vi "Dead Reckoning.vi"(8 "Path":dbl[](array[numeric]), 9 "Yaw angle":dbl, 10 "Channel 6 position":u8, 11 "Velocity":dbl) -> (0 "Yaw with offset":dbl, 1 "Reference yaw":dbl, 2 "Run dead reckoning?":bool, 3 "Reference lean":dbl, 4 "case":dbl)   [LabVIEW 2016]
uses:
  <vilib>/Simulation/Shared/_Datatypes/SIM SISO Transfer Function.ctl
  <vilib>/Simulation/DiscreteLinear/Implementation/NILVSim Discrete Transfer Function Direct.llb/SIM Discrete Transfer Function Diagram (SISO).vi
  <vilib>/Simulation/ContinuousLinear/Implementation/Shared/SIM Transfer Function Support.llb/SIM TransferFunction Normalize to Buffer.vi
  <vilib>/Simulation/DiscreteLinear/Implementation/Shared/SIM Init Discrete States.vi
  <vilib>/Simulation/DiscreteLinear/Implementation/NILVSim Discrete Transfer Function Direct.llb/SIM Transfer Function Direct core (SISO).vi
  <vilib>/Simulation/ContinuousLinear/Implementation/Shared/SIM Transfer Function Support.llb/SIM TransferFunction Normalize.vi
  <vilib>/Simulation/Implementation/Shared/SIM Polynomials.llb/SIM Remove Zero Coefficients (DBL).vi
  <vilib>/Simulation/Implementation/Shared/SIM Polynomials.llb/SIM Divide Polynomials (DBL).vi
  <vilib>/Simulation/Implementation/Shared/SIM BuildSimErr.vi
  <vilib>/Simulation/Implementation/XNodeFramework/SimXNode/SimX.xnode
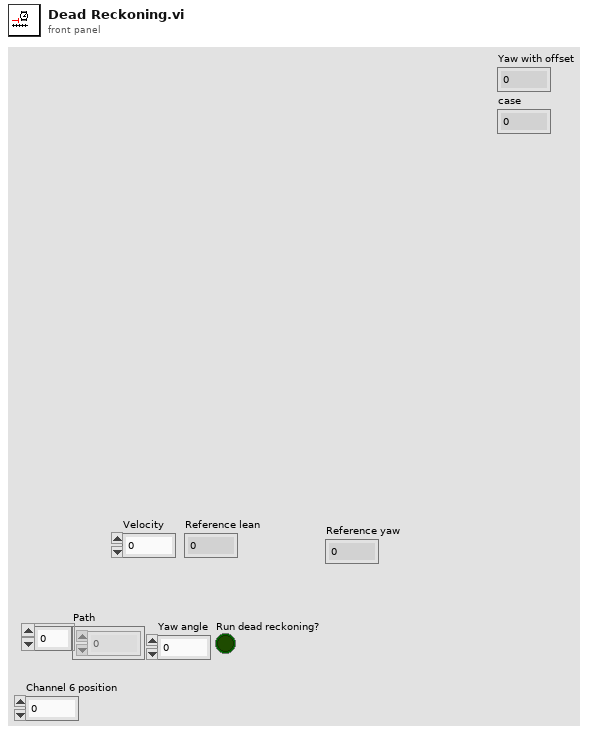
[diagram p1: front panel]
types:
  T1 = cluster{"proportional gain (Kc)":dbl, "integral time (Ti, min)":dbl, "derivative time (Td, min)":dbl}
  T2 = typedef "SIM SISO Transfer Function.ctl" = cluster{"Numerator":dbl[], "Denominator":dbl[]}
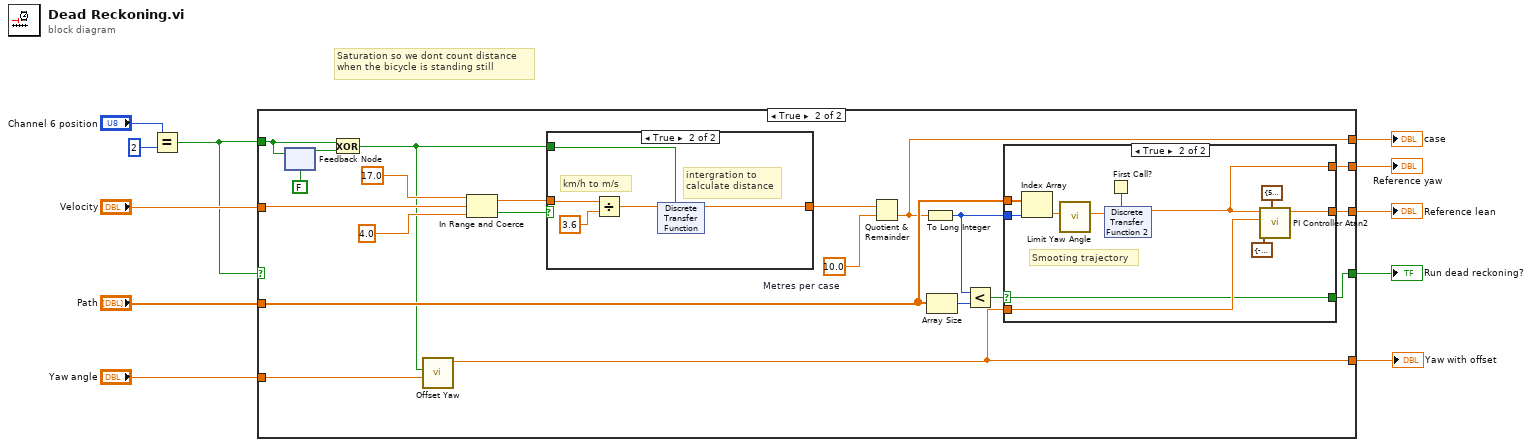
[diagram p0: block diagram]
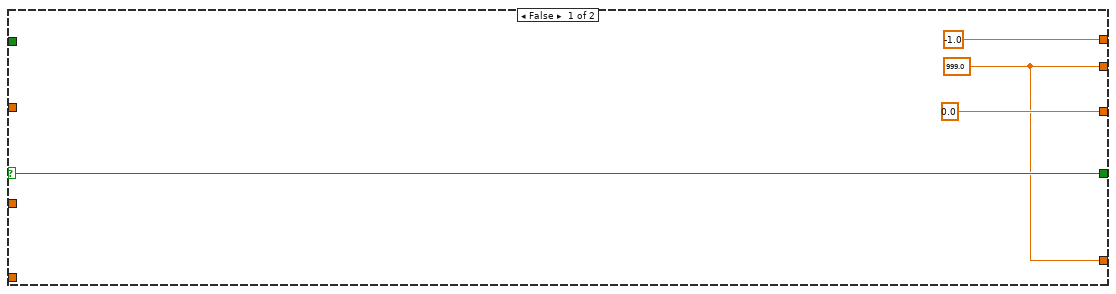
[diagram p2: hidden frame]
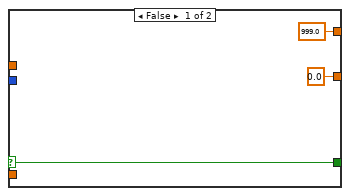
[diagram p3: hidden frame]
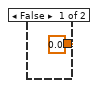
[diagram p4: hidden frame]
diagram:
  # "Saturation so we dont count distance\nwhen the bicycle is standing still"
  n1 = Equal?(x="Channel 6 position", y=u8 2) -> (x = y?=w4:bool)
  n2 = case shown="True" w4 {
    selector: w4 -> [w13 _]
    tunnel: w4 -> [_ w25]
    tunnel: "Velocity" -> [_ w28]
    tunnel: "Path" -> [_ w27]
    tunnel: "Yaw angle" -> [_ w21]
    tunnel: [0.0 ("output") w26] -> w6
    tunnel: [w12 w20] -> w5
    tunnel: [-1.0 w16] -> w3
    tunnel: [w12 w18] -> w2
    tunnel: [w13 w17] -> w1
    frame False {
      w12 = 999.0 ("output y(k)")
    }
    frame True {
      w19 = 10.0  # Metres per case
      n3 = feedback #1(FALSE) -> (w32:bool)
      n4 = feedback-in #1(w25) -> ()
      n5 = Exclusive Or(1:w32, 2:w25) -> (0:w22:bool)
      n6 = call "Offset Yaw.vi"("Sensor Yaw"=w21, "Trigger offset"=w22) -> ("Yaw with offset"=w20:dbl)  [unwired: 9 in]
      n7 = In Range and Coerce(upper limit=17.0, x=w28, lower limit=4.0) -> (coerced(x)=w33:dbl, In Range?=w34:bool)
      n8 = case shown="True" w34 {
        tunnel: w33 -> [_ w61]
        tunnel: w22 -> [_ w59]
        tunnel: [0.0 w58] -> w30
        frame False {
        }
        frame True {
          # "intergration to \ncalculate distance"
          # "km/h to m/s"
          n9 = Divide(x=w61, y=3.6) -> (x/y=w60:dbl)
          n10 = xnode "Discrete Transfer Function"("input u(k)"=w60, "initialize"=w59) -> ("output y(k)"=w58:dbl)  [unwired: 1 in, 1 out]
        }
      }
      n11 = Quotient & Remainder(x=w30, y=w19) -> (floor(x/y)=w16:dbl)  [unwired: 1 out]
      n12 = To Long Integer(number=w16) -> (32bit integer=w23:i32)
      n13 = Array Size(array=w27) -> (size(s)=w29:i32)
      n14 = Less?(x=w23, y=w29) -> (x < y?=w24:bool)
      n15 = case shown="True" w24 {
        selector: w24 -> [w37 w40]
        tunnel: w23 -> [_ w50]
        tunnel: w27 -> [_ w49]
        tunnel: w20 -> [_ w45]
        tunnel: [0.0 ("output") w42] -> w26
        tunnel: [999.0 ("output y(k)") w41] -> w18
        tunnel: [w37 w40] -> w17
        frame False {
        }
        frame True {
          # "Smooting trajectory"
          n16 = Index Array(array=w49, index=w50) -> (element=w48:dbl)
          n17 = call "Limit Yaw Angle.vi"("u"=w48) -> ("output"=w47:dbl)  [unwired: 10 in]
          n18 = First Call?() -> (First Call?: T/F=w46:bool)
          n19 = xnode ("Discrete Transfer Function 2")("input u(k)"=w47, "initialize"=w46) -> ("output y(k)"=w41:dbl)  [unwired: 1 in, 1 out]
          n20 = call "PI Controller Atan2.vi"("output range"=cluster{"output high":dbl, "output low":dbl} {"output high"=5.0, "output low"=-5.0}, "PID gains"=T1 {"proportional gain (Kc)"=-0.07592, "integral time (Ti, min)"=157.202, "derivative time (Td, min)"=0.0}, "process variable"=w45, "setpoint"=w41) -> ("output"=w42:dbl)  [unwired: 6 in, 1 out]
        }
      }
    }
  }
  "Reference lean" <- w6
  "Run dead reckoning?" <- w1
  "Reference yaw" <- w2
  "Yaw with offset" <- w5
  "case" <- w3
